vi "sub_plot_all_channels.vi"(0 "Is first?":bool=TRUE, 1 "Channels":refnum<vi>, 2 "Total current":refnum<vi>, 7 "Plot cluster":T1, 11 "Cluster":cluster{dbl[], dbl[], dbl[]}, 12 "Custom channel":i32, 13 "Total current":dbl, 14 "Data":dbl) -> (8 "Plot cluster out":T1, 15 "Cluster out":cluster{dbl[], dbl[], dbl[]})   [LabVIEW 2016]
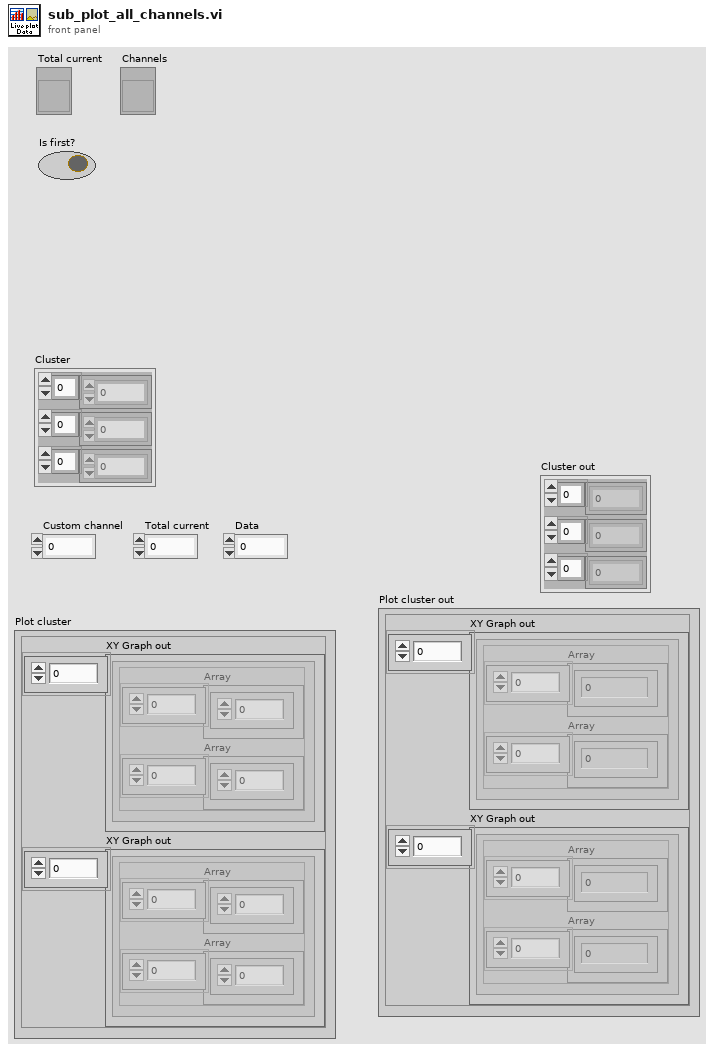
[diagram p1: front panel]
types:
  T1 = cluster{"XY Graph out":cluster{"Array":dbl[], "Array":dbl[]}[], "XY Graph out":cluster{"Array":dbl[], "Array":dbl[]}[]}
  T2 = cluster{"Y array out":dbl[], "X array out":dbl[], "Y array out":dbl[]}
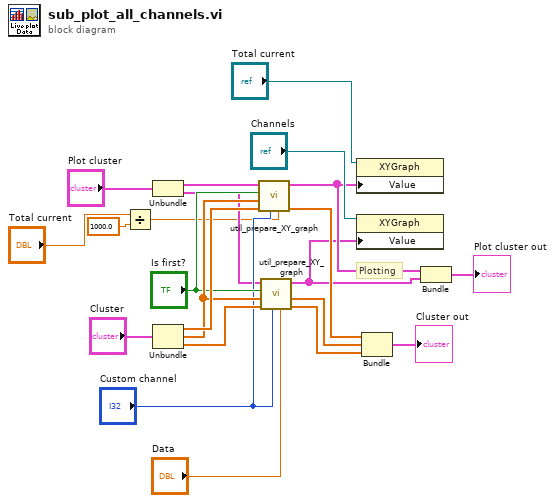
[diagram p0: block diagram]
diagram:
  # "Plotting"
  n1 = Divide(x="Total current", y=1000.0) -> (x/y=w1:dbl)
  n2 = Unbundle("Plot cluster") -> ("XY Graph out"=w5:cluster{"Array":dbl[], "Array":dbl[]}[], "XY Graph out"=w4:cluster{"Array":dbl[], "Array":dbl[]}[])
  n3 = Unbundle("Cluster") -> (w22:dbl[], w21:dbl[], w20:dbl[])
  n4 = call "util_prepare_XY_graph.vi"("Y"=w1, "X"="Custom channel", "Y array"=w22, "X array"=w21, "IsFirst"="Is first?", "XY Graph in"=w5) -> ("Y array out"=w17:dbl[], "XY Graph out"=w9:cluster{"Array":dbl[], "Array":dbl[]}[])  [unwired: 3 in, 1 out]
  n5 = call "util_prepare_XY_graph.vi"("Y"="Data", "X"="Custom channel", "Y array"=w20, "X array"=w21, "IsFirst"="Is first?", "XY Graph in"=w4) -> ("Y array out"=w19:dbl[], "X array out"=w18:dbl[], "XY Graph out"=w8:cluster{"Array":dbl[], "Array":dbl[]}[])  [unwired: 3 in]
  n6 = property class="XYGraph"(reference="Total current", "Value"=w9) -> ()  [unwired: 1 in, 2 out]
  n7 = property class="XYGraph"(reference="Channels", "Value"=w8) -> ()  [unwired: 1 in, 2 out]
  n8 = Bundle("Y array out"=w17, "X array out"=w18, "Y array out"=w19) -> (→"Cluster out":T2)  [unwired: 1 in]
  n9 = Bundle("XY Graph out"=w9, "XY Graph out"=w8) -> (→"Plot cluster out":T1)  [unwired: 1 in]
